vi "DeletePanel.vi"(8 "error in":errorcluster caption="错误输入（无错误）", 11 "PanelRootNode 输入":refnum<class "PanelRootNode.lvclass"> caption="DNL_LabVIEW Object in") -> (0 "error out":errorcluster caption="错误输出", 3 "PanelRootNode 输出":refnum<class "PanelRootNode.lvclass"> caption="DNL_LabVIEW Object out")   [LabVIEW 2013, in "PanelRootNode.lvclass"]
uses:
  PanelRootNode.lvclass
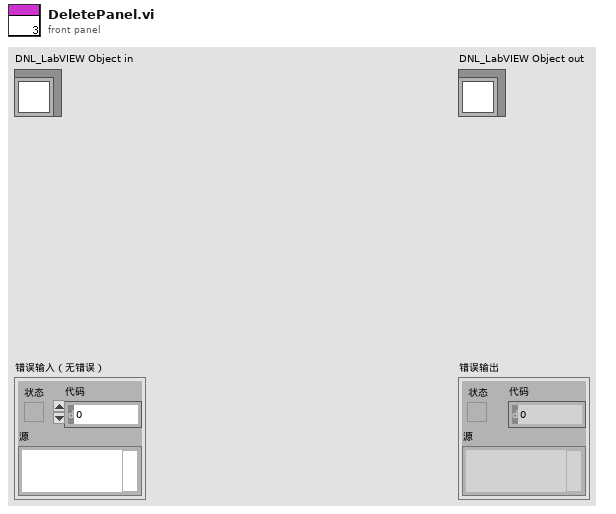
[diagram p1: front panel]
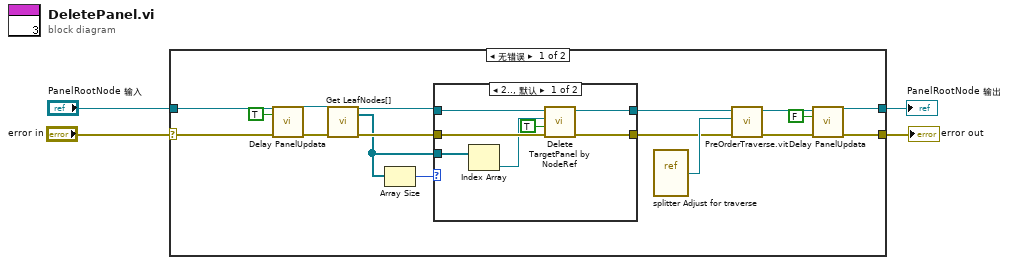
[diagram p0: block diagram]
diagram:
  n1 = case shown="无错误" "error in" {
    selector: "error in" -> [w15 w32]
    tunnel: [w12 w32] -> w3
    tunnel: [w14 w31] -> w1
    tunnel: "PanelRootNode 输入" -> [w18 w31]
    frame No Error {
      n2 = call "Delay PanelUpdata.vi"("error in (no error)"=w15, "延迟前面板更新"=TRUE, "PanelRootNode 输入"=w18) -> ("error out"=w19:errorcluster, "PanelRootNode 输出"=w20:refnum<class "PanelRootNode.lvclass">)  [unwired: 7 in]
      n3 = call "Get LeafNodes[].vi"("error in (no error)"=w19, "PanelRootNode 输入"=w20) -> ("error out"=w16:errorcluster, "LeafNodes[]"=w10:refnum<data-value>[], "PanelRootNode 输出"=w17:refnum<class "PanelRootNode.lvclass">)  [unwired: 7 in]
      n4 = Array Size(array=w10) -> (size(s)=w11:i32)
      n5 = case shown="2.., 默认" w11 {
        tunnel: w17 -> [w28 w30]
        tunnel: w16 -> [w27 w29]
        tunnel: [w26 w30] -> w8
        tunnel: [w25 w29] -> w6
        tunnel: w10 -> [w24 _]
        frame 2.., Default {
          n6 = Index Array(array=w24) -> (element=w23:refnum<data-value>)  [unwired: 1 in]
          n7 = call-dynamic "Delete TargetPanel by NodeRef.vi"("error in"=w27, "Abort VI"=TRUE, "Node*"=w23, "PanelRootNode 输入"=w28) -> ("error out"=w25:errorcluster, "PanelRootNode 输出"=w26:refnum<class "PanelRootNode.lvclass">)  [unwired: 6 in]
        }
        frame 1 {
          # "只有一个面板时不允许删除"
        }
      }
      n8 = vi-ref "splitter Adjust for traverse.vi"() -> (w9:refnum<vi>)
      n9 = call-dynamic "PreOrderTraverse.vit"("error in"=w6, "vi reference"=w9, "PanelLinkNode 输入"=w8) -> ("error out"=w5:errorcluster, "PanelLinkNode 输出"=w7:refnum<class "PanelRootNode.lvclass">)  [unwired: 5 in, 2 out]
      n10 = call "Delay PanelUpdata.vi"("error in (no error)"=w5, "延迟前面板更新"=FALSE, "PanelRootNode 输入"=w7) -> ("error out"=w12:errorcluster, "PanelRootNode 输出"=w14:refnum<class "PanelRootNode.lvclass">)  [unwired: 7 in]
    }
    frame Error {
    }
  }
  "error out" <- w3
  "PanelRootNode 输出" <- w1
